vi "Open New File.vi"(7 "File Path in":path, 8 "error in (no error)":errorcluster, 11 "Data In":T1) -> (0 "error out":errorcluster, 3 "Data Out":T1)   [LabVIEW 2011, in "TDMS Custom Device.lvlib"]
uses:
  TDMS Custom Device.lvlib
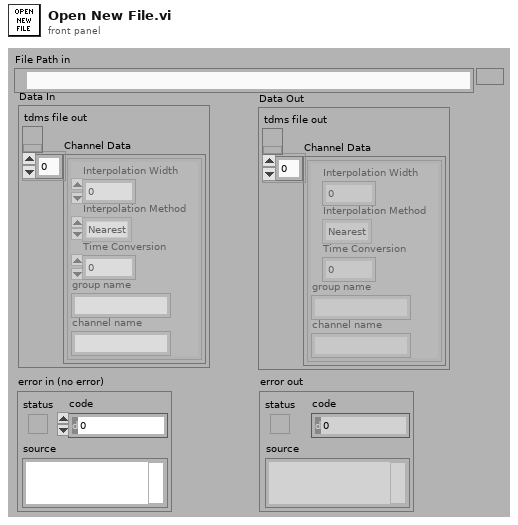
[diagram p1: front panel]
types:
  T1 = cluster{"tdms file out":refnum<k34>, "Channel Data":cluster{"Interpolation Width":i32, "Interpolation Method":enum16{"Nearest", "Linear", "Spline", "Cubic Hermite", "Lagrange", "Polynomial"}, "Time Conversion":dbl, "group name":string, "channel name":string}[]}
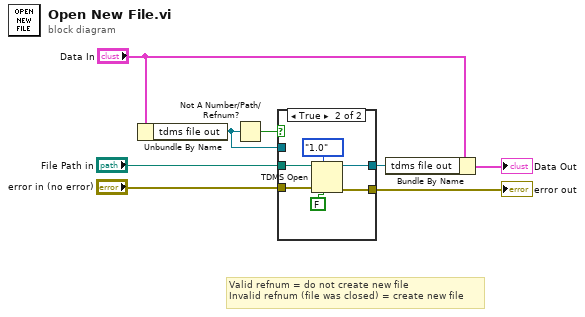
[diagram p0: block diagram]
diagram:
  # "Valid refnum = do not create new file\nInvalid refnum (file was closed) = create new file"
  n1 = Unbundle By Name("Data In") -> ("tdms file out"=w3:refnum<k34>)
  n2 = Not A Number/Path/Refnum?(number/path/refnum=w3) -> (NaN/Path/Refnum?=w4:bool)
  n3 = case shown="True" w4 {
    tunnel: "File Path in" -> [_ w14]
    tunnel: [w9 w13] -> w1
    tunnel: [w10 w12] -> w7
    tunnel: "error in (no error)" -> [w10 w11]
    tunnel: w3 -> [w9 _]
    frame False {
    }
    frame True {
      n4 = TDMS Open(6:FALSE ("disable buffering (T)"), 7:enum16{"1.0", "2.0"}."1.0" ("file format version (2.0)"), 8:w11, 11:w14) -> (0:w12:errorcluster, 3:w13:refnum<k34>)  [unwired: 2 in]
    }
  }
  "error out" <- w7
  n5 = Bundle By Name(cluster="Data In", "tdms file out"=w1) -> (→"Data Out":T1)
